vi "Eject Coin.vi"(0 "reference in":refnum<class "Has Coin State.lvclass">, 5 "error in (no error)":errorcluster) -> (14 "reference out":refnum<class "Has Coin State.lvclass">, 19 "error out":errorcluster)   [LabVIEW 2013, in "Has Coin State.lvclass"]
uses:
  Has Coin State.lvclass
  Gum Machine_class/Gum Machine.lvclass
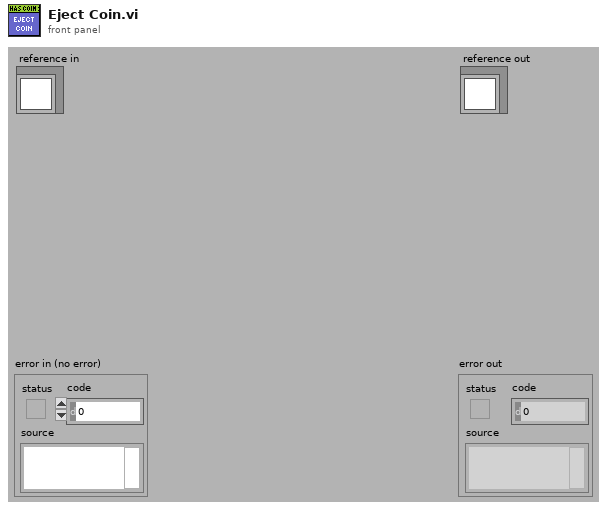
[diagram p1: front panel]
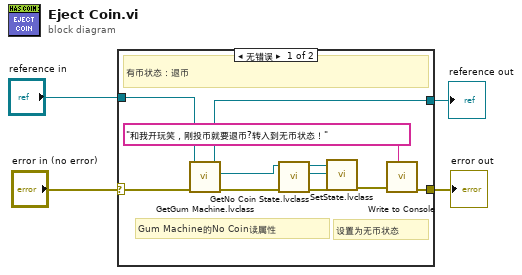
[diagram p0: block diagram]
diagram:
  n1 = case shown="无错误" "error in (no error)" {
    selector: "error in (no error)" -> [w10 w17]
    tunnel: [w15 w17] -> w3
    tunnel: [w9 w16] -> w1
    tunnel: "reference in" -> [w13 w16]
    frame No Error {
      # "设置为无币状态"
      # "Gum Machine的No Coin读属性"
      # "有币状态：退币"
      n2 = call-dynamic "GetGum Machine.lvclass.vi"("error in (no error)"=w10, "reference in"=w13) -> ("error out"=w11:errorcluster, "Gum Machine.lvclass"=w12:refnum<class "Gum Machine.lvclass">, "reference out"=w9:refnum<class "Has Coin State.lvclass">)  [unwired: 7 in]
      n3 = call-dynamic "GetNo Coin State.lvclass.vi"("error in (no error)"=w11, "reference in"=w12) -> ("error out"=w6:errorcluster, "No Coin State.lvclass"=w7:refnum<class "No Coin State.lvclass">, "reference out"=w8:refnum<class "Gum Machine.lvclass">)  [unwired: 7 in]
      n4 = call-dynamic "SetState.lvclass.vi"("error in (no error)"=w6, "State.lvclass"=w7, "reference in"=w8) -> ("error out"=w5:errorcluster)  [unwired: 7 in, 1 out]
      n5 = call "Write to Console.vi"("error in (no error)"=w5, "Input"="和我开玩笑，刚投币就要退币?转入到无币状态！") -> ("error out"=w15:errorcluster)  [unwired: 9 in]
    }
    frame Error {
    }
  }
  "error out" <- w3
  "reference out" <- w1
